vi "Dashboard Main.vi"() -> ()   [LabVIEW 2016]
uses:
  <vilib>/Utility/miscctls.llb/LVRowAndColumnTypeDef.ctl
  <vilib>/event_ctls.llb/eventvkey.ctl
  <vilib>/Rock Robotics/Network Tables/NT Read Boolean.vi
  <vilib>/Rock Robotics/Network Tables/NT Read Numeric Array.vi
  <vilib>/Rock Robotics/WPI/Dashboard/WPI_DashboardLogging Global.vi
panel:
  in  "Camera Settings Right":T1={"Frame Rate"=30, "Compression"=30, "Size"=1, "DB Camera Config"=FALSE} {"Frame Rate" scale=1.0..30.0; "Compression" scale=100.0..-1.0; "Size" items=["640x480", "320x240", "160x120"]}
  in  "Camera Name Right":string(combo)="No Camera Selection"
  out "Camera Info":cluster{"Mbps LED":bool, "Mbps":dbl, "fps":dbl} {"fps" format="%#.1g"; "Mbps" format="%#.1g"}
  in  "Camera Settings":T1={"Frame Rate"=30, "Compression"=30, "Size"=1, "DB Camera Config"=FALSE} {"Frame Rate" scale=1.0..30.0; "Compression" scale=100.0..-1.0; "Size" items=["640x480", "320x240", "160x120"]}
  in  "TCP":refnum<k5>
  in  "Rec Mode":enum32{"Stop", "Record", "Playback"}(radio)
  out "Robot IP":string
  out "Image Message":string="Timeout in Camera Communications"
  in  "Dashboard Tab":T2(tab)
  out "Accelerometer Z Axis":dbl
  out "Accelerometer Y Axis":dbl
  out "Accelerometer X Axis":dbl
  out "Vision Align":bool
  out "LEFT SPEED VARIABLE FEEDBACK":dbl
  in  "LEFT SPEED VARIABLE":dbl
  out "RIGHT SPEED VARIABLE FEEDBACK":dbl
  in  "RIGHT SPEED VARIABLE":dbl
  in  "Select Auto":string(combo)="Select Autonomous ..."
  out "NT Connection":bool
  out "MotorChart R":cluster{"Numeric":dbl, "Numeric":dbl}(graph)
  out "MotorChart L":cluster{"Numeric":dbl, "Numeric":dbl}(graph)
  out "MotorSliders R":cluster{"MotorSlide1":dbl, "MotorSlide2":dbl} {"MotorSlide2" scale=-1.0..1.0 scale format="%#_2e"; "MotorSlide1" scale=-1.0..1.0 scale format="%#_2e"}
  out "MotorSliders L":cluster{"MotorSlide1":dbl, "MotorSlide2":dbl} {"MotorSlide2" scale=-1.0..1.0 scale format="%#_2e"; "MotorSlide1" scale=-1.0..1.0 scale format="%#_2e"}
  out "Gyro":dbl(knob) scale=0.0..360.0
  out "JS1 Z":dbl(slide) scale=-1.0..1.0 scale format="%#_2e"
  out "JS1 Graph":cluster{"X":dbl, "Y":dbl}[](graph)
  out "JS1 Buttons":T3
  out "JS2 Z":dbl(slide) scale=-1.0..1.0 scale format="%#_2e"
  out "JS2 Graph":cluster{"X":dbl, "Y":dbl}[](graph)
  out "JS2 Buttons":T3
  out "Mode":T4(ring)=enum."Auto Disabled"
  out "RightMotors":dbl
  out "LeftMotors":dbl
  out "Right Y Axis":dbl
  out "Right X Axis":dbl
  out "Left X Axis":dbl
  out "Left Y Axis":dbl
  out "Vision Nothing In Sight":bool
  out "Camera Image Right":T5(plugin-control)
  out "X Average":dbl
  out "Vision Align 2":bool
  in  "DB/String 9":string
  in  "DB/String 8":string
  in  "DB/String 7":string
  in  "DB/String 6":string
  in  "DB/String 5":string
  in  "DB/String 4":string
  in  "DB/String 3":string
  in  "DB/String 2":string
  in  "DB/String 1":string
  in  "DB/String 0":string
  in  "DB/Slider 0":dbl(slide) scale=0.0..5.0
  in  "DB/Slider 1":dbl(slide) scale=0.0..5.0
  in  "DB/Slider 2":dbl(slide) scale=0.0..5.0
  in  "DB/Slider 3":dbl(slide) scale=0.0..5.0
  out "DB/LED 3":bool
  out "DB/LED 2":bool
  out "DB/LED 1":bool
  out "DB/LED 0":bool
  in  "DB/Button 3":bool
  in  "DB/Button 2":bool
  in  "DB/Button 1":bool
  in  "DB/Button 0":bool caption="New Name"
  out "Autonoums Delay FEEDBACK":dbl
  in  "Autonoums Delay":dbl
  out "Vision align Range correction VARIABLE FEEDBACK":dbl
  in  "Vision align Range correction VARIABLE":dbl
  out "Vision align Oscillation correction VARIABLE FEEDBACK":dbl
  in  "Vision align Oscillation correction VARIABLE":dbl
  out "Periodic Gyro forward SPEED VARIABLE FEEDBACK":dbl
  in  "Periodic Gyro forward SPEED VARIABLE":dbl
  out "Autonomos Gyro forward SPEED VARIABLE FEEDBACK":dbl
  in  "Autonomos Gyro forward SPEED VARIABLE":dbl
  in  "Test Slider":dbl(slide) scale=0.0..100.0 scale format="%#_3g"
  in  "On/Off":bool caption="Solenoid"
  in  "Test Name":u16(ring) items=["Select the test to run..."]
  in  "Test Tree":string(tree)
  in  "Motor":cluster{"Value":dbl, "Enable":bool} {"Value" scale=-1.0..1.0 scale format="%#_3g"}
  out "Progress":T6 {"Test Progress" scale=0.0..100.0}
  in  "Rev/Fwd":cluster{"Forward":bool, "Reverse":bool}
  in  "Test Ring":u16(ring) items=["Monochrome", "Color"]
  out "Cmd Status":string
  in  "Execute Command":bool
  in  "Command Params":string[][](table)
  in  "Command Selection":i32(listbox)
  in  "CheckList":i32(listbox)
  out "Tree":string(tree)
  out "Camera Image":T5(plugin-control)
  out "Background":bool
  in  "Camera Name":string(combo)="No Camera Selection"
  # "HW"
  # "HW"
  # "Joysticks"
  # "Drive Motors"
  # "Front"
  # "Right"
  # "Left"
  # "Back"
  # "Should be 0.4"
  # "Should be 0.3"
  # "Should be 0.45"
  # "Should be 0.5"
  # "Should be 0.2"
  # "Should be 0.1"
  # "Should be 1500"
  # "This tab is a great place for autonomous settings and robot-specific values.\nPlace controls and indicators inside this tab and match name to\nDashboard Variables on robot. You can also delete this comment."
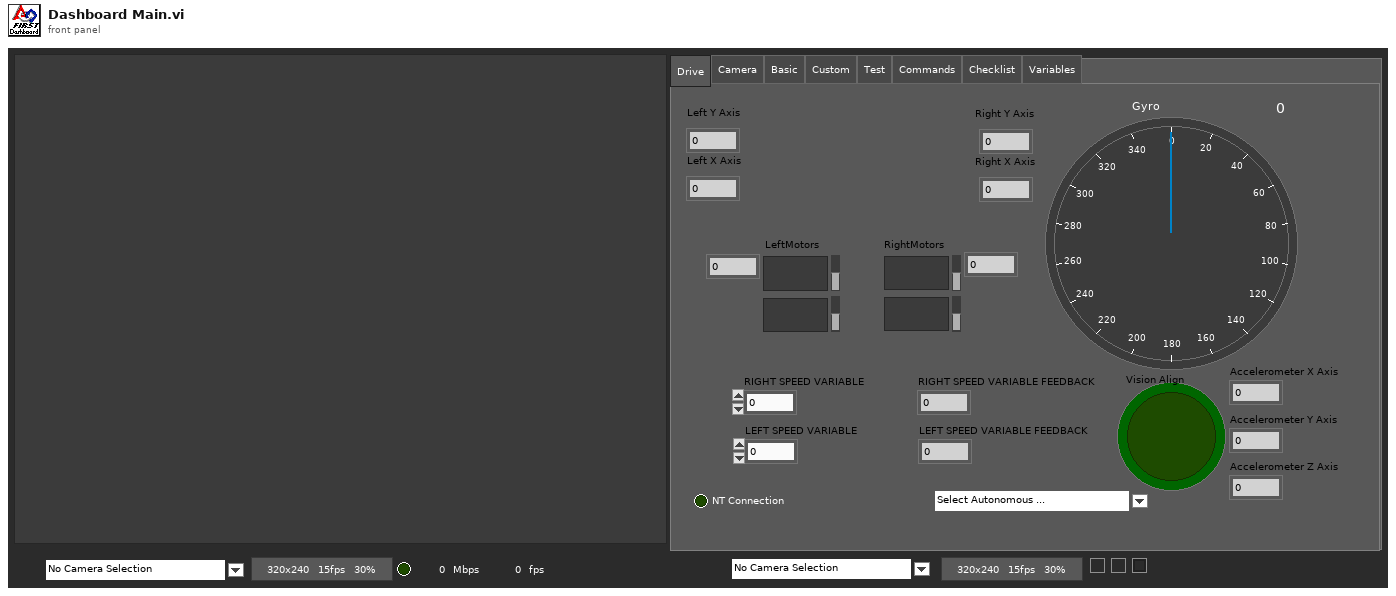
[diagram p1: front panel]
types:
  T1 = cluster{"Frame Rate":i32, "Compression":i32, "Size":u16, "DB Camera Config":bool}
  T2 = enum32{"Drive", "Camera", "Basic", "Custom", "Test", "Commands", "Checklist", "Variables"}
  T3 = cluster{bool, bool, bool, bool, bool, bool, bool, bool, bool, bool, bool, bool}
  T4 = enum8{"Tele-Op Disabled", "Tele-Op Enabled", "Auto Disabled", "Auto Enabled", "Test Disabled", "Test Enabled", "Disconnected", "No Code", "E-Stop"}
  T5 = typedef "IMAQ Image.ctl" = refnum<image>
  T6 = cluster{"Test Progress":u8, "Test Progress Text":string}
  T7 = typedef "Image Type" = u32
  T8 = cluster{"IDs":cluster{"RPC field ID":u16, "Unique ID":u16}, "String":string}
  T9 = enum32{"Drive", "Basic", "Custom", "Test", "Checklist", "Variables"}
  T10 = cluster{"Error Strings":string, "Disable Counts":cluster{u16, u16}, "Rail Faults":cluster{u16, u16, u16}, "Robot IP":string, "DB Mode":u8, "Event Info":cluster{"Name":string, "Type":u8, "Number":u16, "Replay":u8}}
  T11 = cluster{"Storage":cluster{"Disk Free":u64, "RAM Block":u32, "RAM free":u32}, "CPU Utilization":cluster{"CPU % ISR":sgl, "CPU % Time Crit":sgl, "CPU % Timed Str":sgl, "CPU % High":sgl, "CPU % Above":sgl, "CPU % Normal":sgl, "CPU % Low":sgl}, "CAN":cluster{"% Bus Utilization":sgl, "Bus Off Cnt":u32, "TX_FIFO Full Cnt":u32, "Receive Error Cnt":u8, "Transmit Error Cnt":u8}, "HID":cluster{"HID Outputs":u32, "Rumble Low":u16, "Rumble High":u16}[]}
  T12 = cluster{"Status bits":cluster{"Test Mode":bool, "Autonomous":bool, "Enabled":bool, "Code Start":bool, "Brownout":bool, "Reserved 2":bool, "Reserved 3":bool, "E-Stop":bool}, "Code Trace":cluster{"Disabled":bool, "TeleOp":bool, "Auto":bool, "Test":bool}, "Controller Type":enum16{"unknown", "cRIO", "roboRio"}, "Code?":enum16{"unknown", "noCode", "code"}, "Battery V":dbl}
  T13 = cluster{"Control Bits":cluster{"TestMode":bool, "Autonomous":bool, "Enabled":bool, "FMS Present":bool, bool, bool, bool, "E-Stop":bool}, "Team Station ":u8, "Countdown":sgl, "Joystick Values":cluster{"Axes":dbl[], "Buttons":bool[], "POVs":i16[]}[]}
  T14 = cluster{"Axes":dbl[], "Buttons":bool[], "POVs":i16[]}[]
  T15 = cluster{"Axes":dbl[], "Buttons":bool[], "POVs":i16[]}
  T16 = cluster{"Buttons[0]":bool, "Buttons[1]":bool, "Buttons[2]":bool, "Buttons[3]":bool, "Buttons[4]":bool, "Buttons[5]":bool, "Buttons[6]":bool, "Buttons[7]":bool, "Buttons[8]":bool, "Buttons[9]":bool, "Buttons[10]":bool, "Buttons[11]":bool}
  T17 = cluster{"Camera Image":refnum<vi>, "Dashboard Tab":refnum<vi>, "Background":refnum<vi>, "Rec Mode":refnum<vi>, "Test Slider":refnum<vi>, "On/Off ":refnum<vi>, "Test Ring":refnum<vi>, "Rev/Fwd":refnum<vi>, "Test Name":refnum<vi>, "Motor":refnum<vi>, "Progress":refnum<vi>, "CheckList":refnum<vi>, "Tree":refnum<vi>, "Test Tree":refnum<vi>, "Command Params":refnum<vi>, "Command Selection":refnum<vi>, "Execute Command":refnum<vi>, "Cmd Status":refnum<vi>, "Camera Settings":refnum<vi>, "Camera Name":refnum<vi>, "Camera Info":refnum<vi>, "Camera Settings Right":refnum<vi>, "Camera Name Right":refnum<vi>, "Camera Image Right":refnum<vi>}
  T18 = cluster{"Pixels ":cluster{"Start":cluster{"X":dbl, "Y":dbl}, "End":cluster{"X":dbl, "Y":dbl}}, "Real World":cluster{"Start":cluster{"X":dbl, "Y":dbl}, "End":cluster{"X":dbl, "Y":dbl}}}
  T19 = cluster{"Operation":enum16{"Update", "Clear"}, "Color Box":u32}[]
  T20 = typedef "eventvkey.ctl" = enum16{"ASCII", "Enter", "Return", "Shift", "Ctrl", "Alt", "Cmd", "Opt", "Caps", "NumLock", "Clear", "Break", "Up", "Down", "Left", "Right", "Insert", "Delete", "Home", "End", "PageUp", "PageDown", "Escape", "Help", "Pause", "ScrollLock", "F1", "F2", "F3", "F4", "F5", "F6", "F7", "F8", "F9", "F10", "F11", "F12", "F13", "F14", "F15", "F16", "F17", "F18", "F19", "F20", "F21", "F22", "F23", "F24", "Play", "VolumeUp", "VolumeDown", "Mute", "Two Byte Char"}
  T21 = cluster{"Image Size":bool, "Image Type":bool, "Pixel Value":bool, "ROI Information":bool, "Zoom Factor":bool}
  T22 = cluster{"Operation":enum16{"Update", "Clear"}, "Color Box":u32}
  T23 = typedef "LVRowAndColumnTypeDef.ctl" = cluster{"Row":i32, "Column":i32}
  T24 = cluster{"Shift":bool, "Ctrl":bool, "Alt":bool, "Cmd":bool, "Opt":bool}
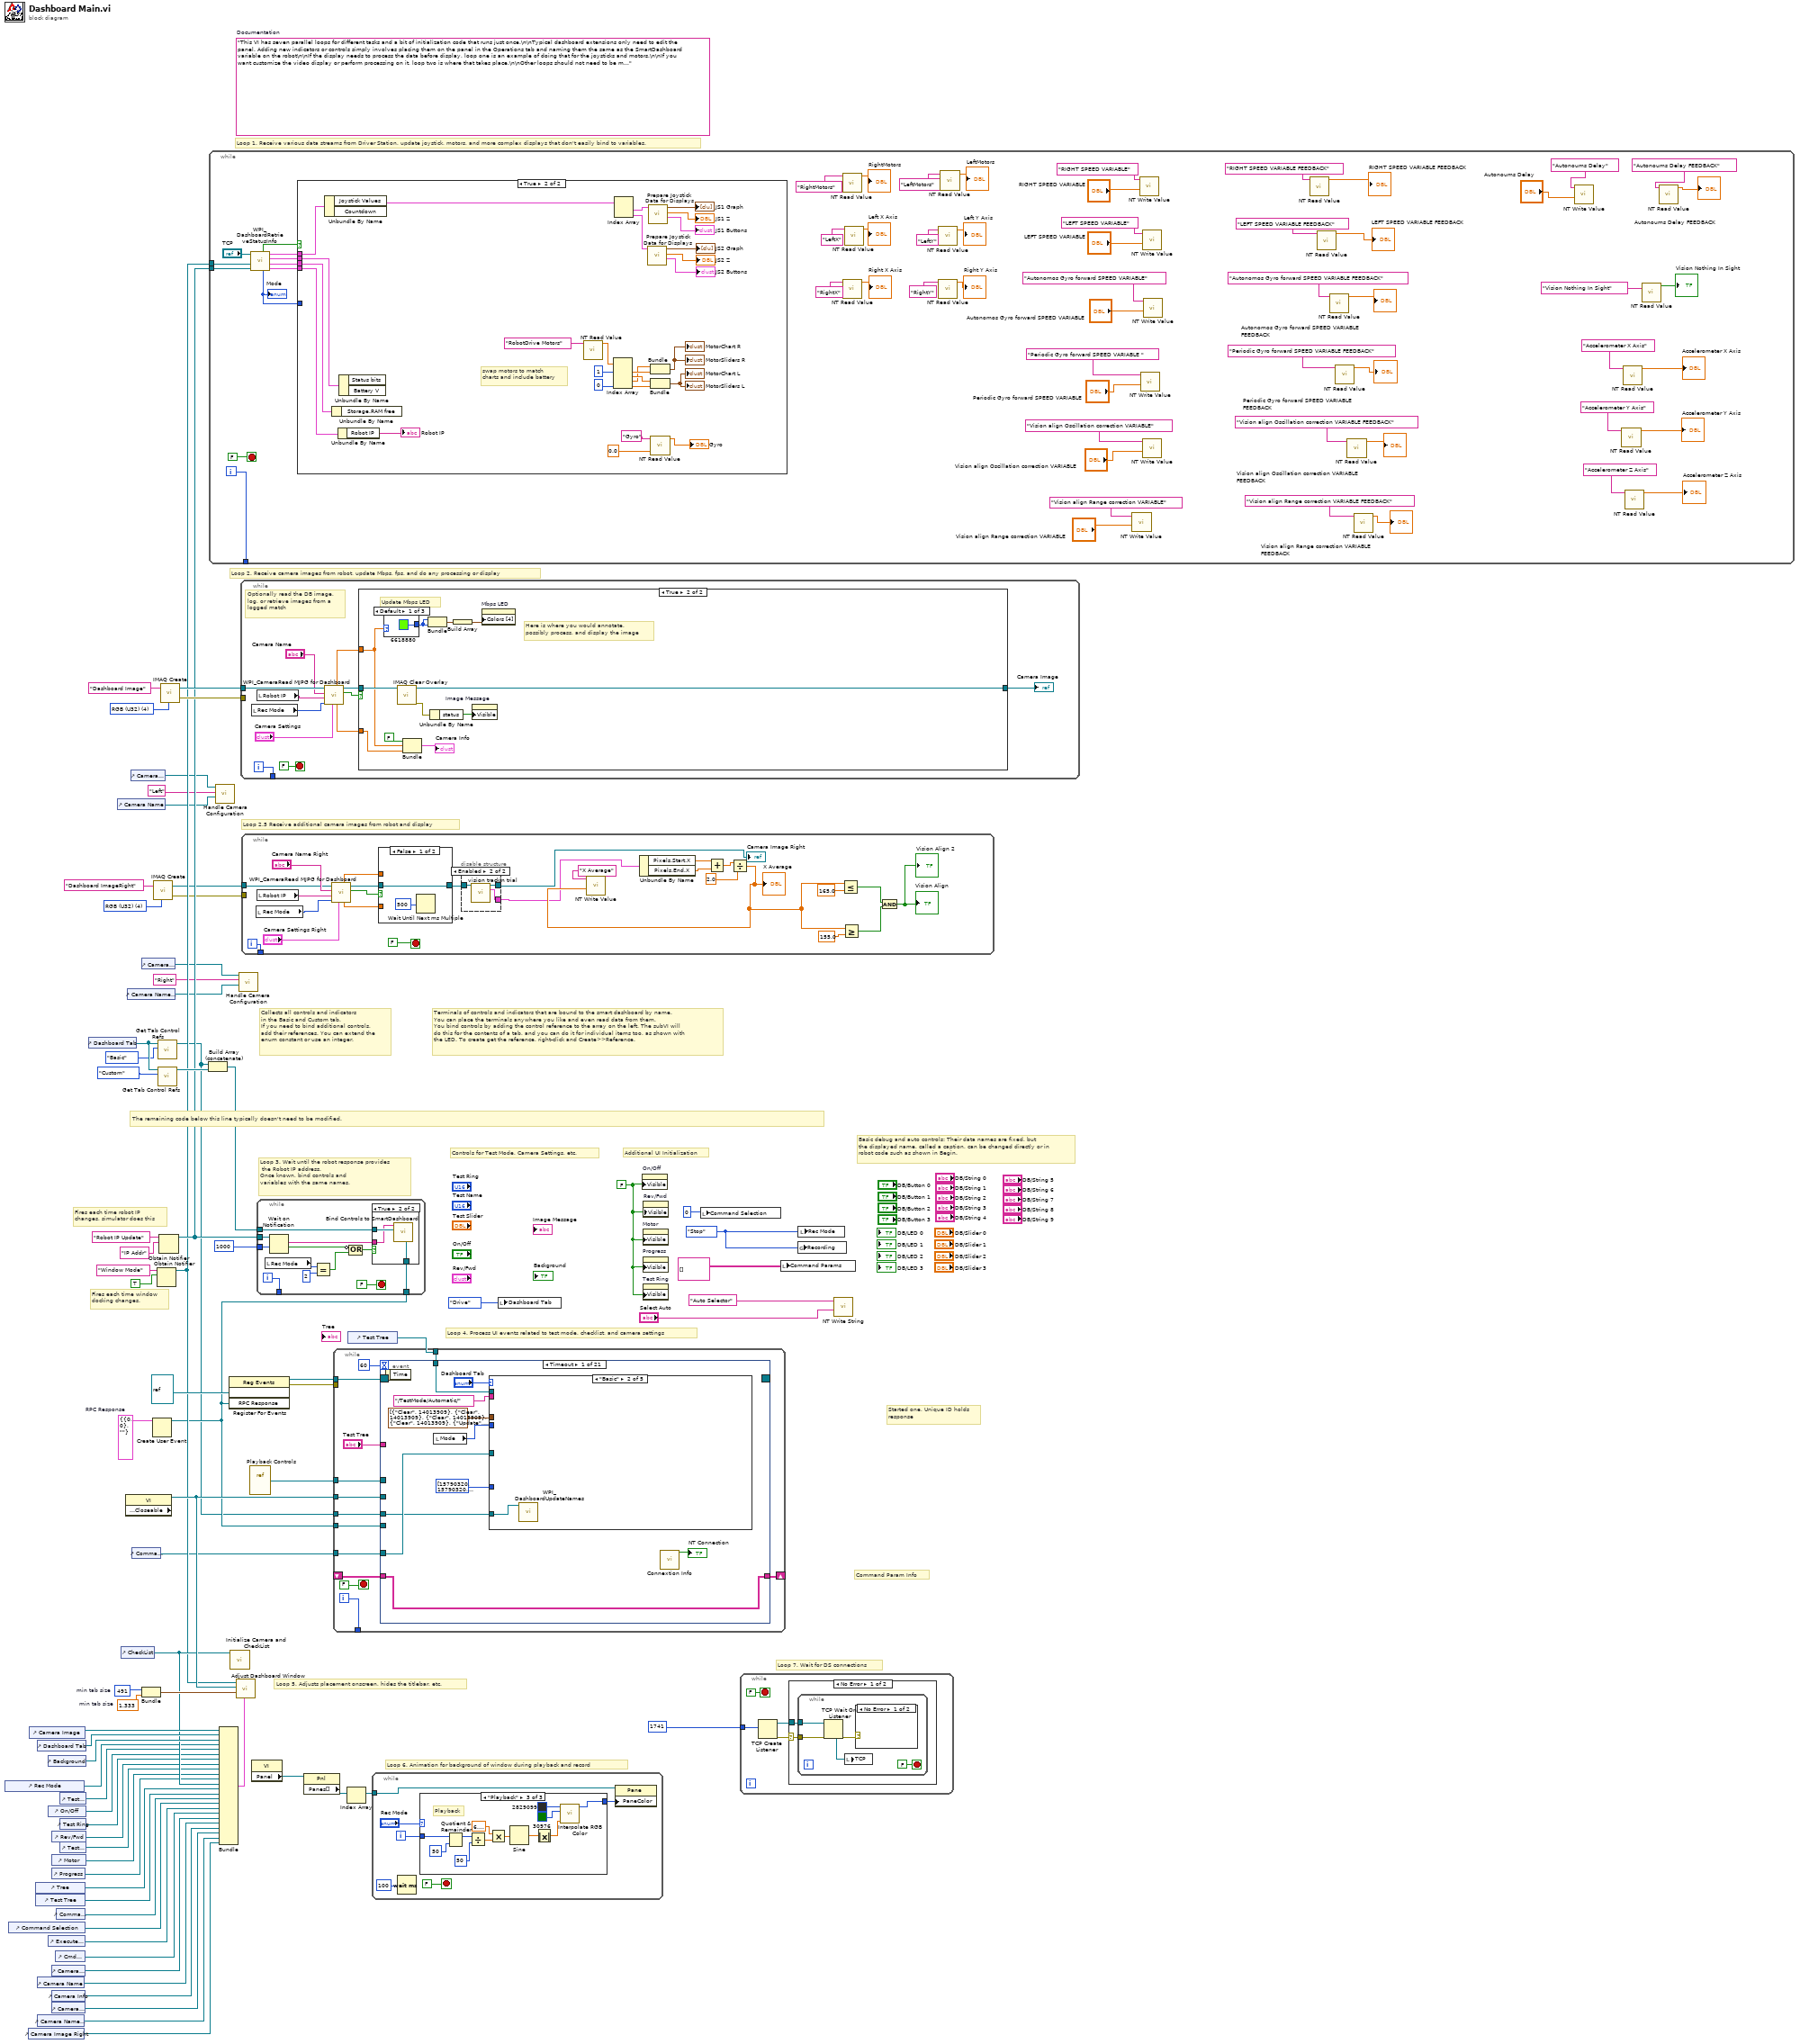
[diagram p0: block diagram]
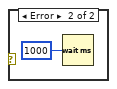
[diagram p4: hidden frame]
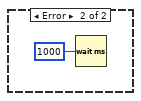
[diagram p5: hidden frame]
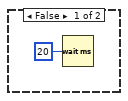
[diagram p6: hidden frame]
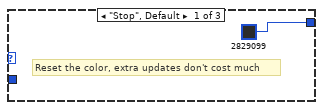
[diagram p7: hidden frame]
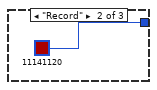
[diagram p8: hidden frame]
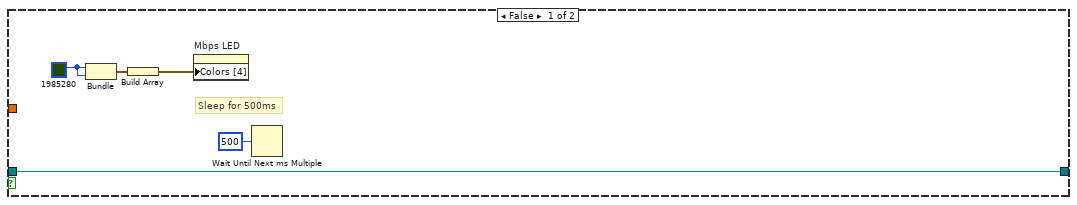
[diagram p10: hidden frame]
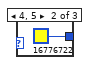
[diagram p11: hidden frame]
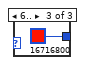
[diagram p12: hidden frame]
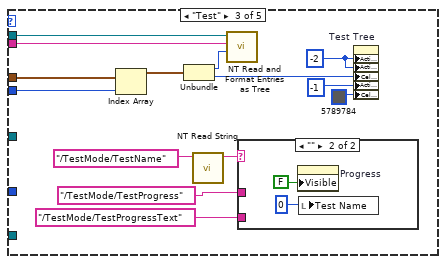
[diagram p14: hidden frame]
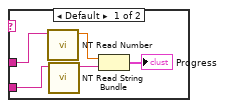
[diagram p15: hidden frame]
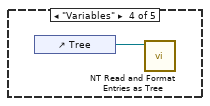
[diagram p16: hidden frame]
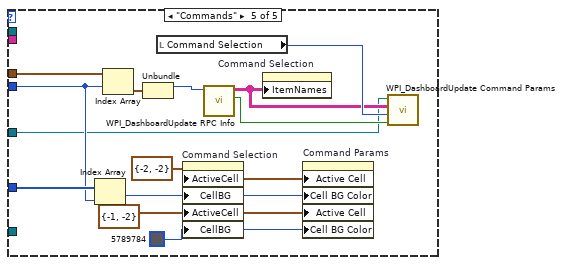
[diagram p17: hidden frame]
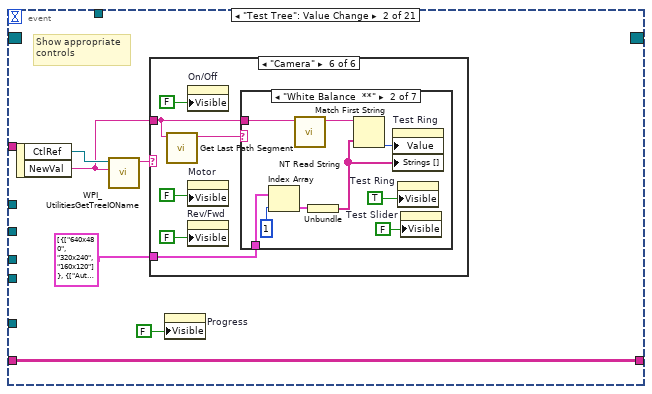
[diagram p18: hidden frame]
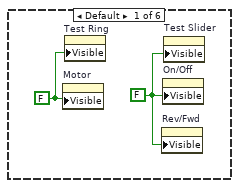
[diagram p19: hidden frame]
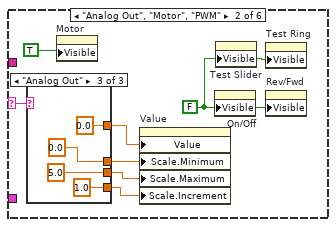
[diagram p20: hidden frame]
diagram:
  w10 = T7 4 items=["Grayscale (U8)", "Grayscale (I16)", "Grayscale (SGL)", "Complex (CSG)", "RGB (U32)", "HSL (U32)", "RGB (U64)"] ("Image Type")
  w26 = T8 {"IDs"={"RPC field ID"=0, "Unique ID"=0}, "String"=""}  # RPC Response
  w51 = 491  # min tab size
  w50 = 1.333  # min tab size
  w58 = enum32{"Stop", "Record", "Playback"}."Stop" ("Rec Mode")
  w33 = FALSE ("Visible")
  (unwired) "This VI has seven parallel loops for different tasks and a bit of initialization code that runs just once.\n\nTypical dashboard extensions only need to edit the panel. Adding new indicators or controls simply involves placing them on the panel in the Operations tab and naming them the same as the SmartDashboard variable on the robot\n\nIf the display needs to process the data before display, loop one is an example of doing that for the joysticks and motors.\n\nIf you want customize the video display or perform processing on it, loop two is where that takes place.\n\nOther loops should not need to be modified. They are pretty standard, and document the task they perform."  # Documentation
  w75 = T7 4 items=["Grayscale (U8)", "Grayscale (I16)", "Grayscale (SGL)", "Complex (CSG)", "RGB (U32)", "HSL (U32)", "RGB (U64)"] ("Image Type")
  # "Loop 2.5 Receive additional camera images from robot and display"
  # "Command Param Info"
  # "Started one, Unique ID holds\nresponse"
  # "Loop 7. Wait for DS connections"
  # "Basic debug and auto controls: Their data names are fixed, but\nthe displayed name, called a caption, can be changed directly or in\nrobot code such as shown in Begin."
  # "Controls for Test Mode, Camera Settings, etc."
  # "Additional UI Initialization"
  # "Loop 6. Animation for background of window during playback and record"
  # "Fires each time robot IP\nchanges, simulator does this"
  # "Fires each time window\ndocking changes."
  # "Collects all controls and indicators\nin the Basic and Custom tab.\nIf you need to bind additional controls,\nadd their references. You can extend the\nenum constant or use an integer."
  # "The remaining code below this line typically doesn't need to be modified."
  # "Loop 4. Process UI events related to test mode, checklist, and camera settings"
  # "Terminals of controls and indicators that are bound to the smart dashboard by name.\nYou can place the terminals anywhere you like and even read data from them.\nYou bind controls by adding the control reference to the array on the left. The subVI will\ndo this for the contents of a tab, and you can do it for individual items too, as shown with\nthe LED. To create get the reference, right-click and Create>>Reference."
  # "Loop 3. Wait until the robot response provides\n the Robot IP address.\nOnce known, bind controls and\nvariables with the same names."
  # "Loop 5. Adjusts placement onscreen, hides the titlebar, etc."
  # "Loop 1. Receive various data streams from Driver Station, update joystick, motors, and more complex displays that don't easily bind to variables."
  # "Loop 2. Receive camera images from robot, update Mbps, fps, and do any processing or display"
  n1 = control-ref of="Rec Mode"() -> (w39:refnum<vi>)
  n2 = control-ref of="Command Selection"() -> (w25:refnum<vi>)
  n3 = control-ref of="Camera Image Right"() -> (w1:refnum<vi>)
  n4 = control-ref of="Camera Image"() -> (w53:refnum<vi>)
  n5 = control-ref of="Tree"() -> (w43:refnum<vi>)
  n6 = control-ref of="Test Tree"() -> (w42:refnum<vi>)
  n7 = control-ref of="Dashboard Tab"() -> (w52:refnum<vi>)
  n8 = control-ref of="Camera Name"() -> (w16:refnum<vi>)
  n9 = control-ref of="Camera Name Right"() -> (w2:refnum<vi>)
  n10 = control-ref of="Execute Command"() -> (w27:refnum<vi>)
  n11 = control-ref of="Background"() -> (w48:refnum<vi>)
  n12 = control-ref of="On/Off"() -> (w37:refnum<vi>)
  n13 = control-ref of="Progress"() -> (w34:refnum<vi>)
  n14 = control-ref of="Camera Settings"() -> (w17:refnum<vi>)
  n15 = control-ref of="Camera Info"() -> (w15:refnum<vi>)
  n16 = control-ref of="Camera Settings Right"() -> (w3:refnum<vi>)
  n17 = control-ref of="Rev/Fwd"() -> (w35:refnum<vi>)
  n18 = control-ref of="Motor"() -> (w40:refnum<vi>)
  n19 = control-ref of="Cmd Status"() -> (w21:refnum<vi>)
  n20 = control-ref of="Command Params"() -> (w28:refnum<vi>)
  n21 = control-ref of="Test Slider"() -> (w38:refnum<vi>)
  n22 = control-ref of="Test Ring"() -> (w36:refnum<vi>)
  n23 = control-ref of="Test Name"() -> (w41:refnum<vi>)
  n24 = control-ref of="Dashboard Tab"() -> (w56:refnum<vi>)
  n25 = control-ref of="Camera Name"() -> (w18:refnum<vi>)
  n26 = control-ref of="CheckList"() -> (w44:refnum<vi>)
  n27 = property class="VI" props=["Front Panel.Closeable"]() -> (reference out=w57:refnum<vi>)  [unwired: 2 in, 2 out]
  n28 = control-ref of="Camera Name Right"() -> (w6:refnum<vi>)
  n29 = control-ref of="Camera Settings"() -> (w19:refnum<vi>)
  n30 = control-ref of="Command Params"() -> (w20:refnum<vi>)
  n31 = control-ref of="Camera Settings Right"() -> (w7:refnum<vi>)
  n32 = Bundle("min tab size"=w51, "min tab size"=w50) -> (w49:cluster{"min tab size":i32, "min tab size":dbl})  [unwired: 1 in]
  n33 = Create User Event(user event datatype=w26) -> (user event=w22:refnum<user-event>)  [unwired: 1 in, 1 out]
  n34 = call "IMAQ Create"("Image Name"="Dashboard ImageRight", "Image Type"=w10) -> ("New Image"=w9:T5, "error out"=w8:errorcluster)  [unwired: 2 in, 1 out]
  n35 = Obtain Notifier(name (unnamed)="Window Mode", notification data type=TRUE) -> (notifier out=w31:refnum<notifier>)  [unwired: 2 in, 2 out]
  n36 = call <vilib>:"Get Tab Control Refs.vi"("Page Index"=T9."Basic" ("Dashboard Tab"), "TabControl in"=w56) -> ("ControlsOnPage"=w14:refnum<vi>[])  [unwired: 9 in]
  n37 = call <vilib>:"Get Tab Control Refs.vi"("Page Index"=T9."Custom" ("Dashboard Tab"), "TabControl in"=w56) -> ("ControlsOnPage"=w55:refnum<vi>[])  [unwired: 9 in]
  n38 = Obtain Notifier(name (unnamed)="Robot IP Update", notification data type="IP Addr" ("name (unnamed)")) -> (notifier out=w32:refnum<notifier>)  [unwired: 2 in, 2 out]
  n39 = call "IMAQ Create"("Image Name"="Dashboard Image", "Image Type"=w75) -> ("New Image"=w73:T5, "error out"=w72:errorcluster)  [unwired: 2 in, 1 out]
  n40 = Build Array (concatenate)(w14, w55) -> (w54:refnum<vi>[])
  n41 = while {
    tunnel: [w133] -> _
    tunnel: w32 -> [w127]
    tunnel: w31 -> [w124]
    i -> [w133]
    stop <- FALSE stop-if-true
    n42 = call <vilib>:"WPI_DashboardRetrieveStatusInfo.vi"("Binding Refnum"=w127, "Window Mode Notifier"=w124, "TCP Cnx"="TCP") -> ("Power and Errors"=w128:T10, "Robot Metrics"=w131:T11, "Status Info"=w132:T12, "Control Info"=w129:T13, "Robot Mode"=w126:T4, "Process?"=w130:bool)  [unwired: 3 in]
    "Mode" <- w126
    n43 = case shown="True" w130 {
      tunnel: w132 -> [_ w162]
      tunnel: w131 -> [_ w161]
      tunnel: w129 -> [_ w160]
      tunnel: w128 -> [_ w159]
      tunnel: w126 -> [_ _]
      frame False {
        n44 = Wait (ms)(milliseconds to wait=u32 20) -> ()  [unwired: 1 out]
      }
      frame True {
        # "swap motors to match\ncharts and include battery"
        n45 = Unbundle By Name(w160) -> ("Joystick Values"=w150:T14)  [unwired: 1 out]
        n46 = Unbundle By Name(w161) -> ()  [unwired: 1 out]
        n47 = Unbundle By Name(w159) -> ("Robot IP"=→"Robot IP":string)
        n48 = Unbundle By Name(w162) -> ()  [unwired: 2 out]
        n49 = call-poly <vilib>:"NT Read Value.vi"("Name"="RobotDrive Motors") -> ("Numeric Array"=w140:dbl[])  [unwired: 9 in, 1 out]
        n50 = Index Array(array=w140, index #1=1, index #4=0) -> (element #1=w154:dbl, element #2=w155:dbl, element #3=w153:dbl, element #4=w158:dbl)  [unwired: 2 in]
        n51 = Index Array(array=w150) -> (element #1=w149:T15, element #2=w145:T15)  [unwired: 2 in]
        n52 = call "Prepare Joystick Data for Displays.vi"("Joystick Values"=w145) -> ("Buttons"=→"JS2 Buttons":T16, "Z Axis"=→"JS2 Z":dbl, "Cartesian Data"=→"JS2 Graph":cluster{"X axis":dbl, "X axis":dbl}[])  [unwired: 8 in]
        n53 = call "Prepare Joystick Data for Displays.vi"("Joystick Values"=w149) -> ("Buttons"=→"JS1 Buttons":T16, "Z Axis"=→"JS1 Z":dbl, "Cartesian Data"=→"JS1 Graph":cluster{"X axis":dbl, "X axis":dbl}[])  [unwired: 8 in]
        n54 = Bundle("Numeric"=w153, "Numeric"=w154) -> (→"MotorChart R" →"MotorSliders R":cluster{"Numeric":dbl, "Numeric":dbl})  [unwired: 1 in]
        n55 = Bundle("Numeric"=w155, "Numeric"=w158) -> (→"MotorChart L" →"MotorSliders L":cluster{"Numeric":dbl, "Numeric":dbl})  [unwired: 1 in]
        n56 = call-poly <vilib>:"NT Read Value.vi"("Default Value"=0.0, "Name"="Gyro") -> ("Numeric"=→"Gyro":dbl)  [unwired: 8 in, 1 out]
      }
    }
    n57 = call-poly <vilib>:"NT Read Value.vi"("Name"="RightMotors") -> ("Numeric"=→"RightMotors":dbl)  [unwired: 9 in, 1 out]
    n58 = call-poly <vilib>:"NT Read Value.vi"("Name"="RightX") -> ("Numeric"=→"Right X Axis":dbl)  [unwired: 9 in, 1 out]
    n59 = call-poly <vilib>:"NT Read Value.vi"("Name"="LeftX") -> ("Numeric"=→"Left X Axis":dbl)  [unwired: 9 in, 1 out]
    n60 = call-poly <vilib>:"NT Read Value.vi"("Name"="LeftY") -> ("Numeric"=→"Left Y Axis":dbl)  [unwired: 9 in, 1 out]
    n61 = call-poly <vilib>:"NT Read Value.vi"("Name"="RightY") -> ("Numeric"=→"Right Y Axis":dbl)  [unwired: 9 in, 1 out]
    n62 = call-poly <vilib>:"NT Read Value.vi"("Name"="LeftMotors") -> ("Numeric"=→"LeftMotors":dbl)  [unwired: 9 in, 1 out]
    n63 = call-poly <vilib>:"NT Write Value.vi"("Numeric"="Vision align Range correction VARIABLE", "Name"="Vision align Range correction VARIABLE") -> ()  [unwired: 9 in, 1 out]
    n64 = call-poly <vilib>:"NT Write Value.vi"("Numeric"="RIGHT SPEED VARIABLE", "Name"="RIGHT SPEED VARIABLE") -> ()  [unwired: 9 in, 1 out]
    n65 = call-poly <vilib>:"NT Write Value.vi"("Numeric"="Periodic Gyro forward SPEED VARIABLE", "Name"="Periodic Gyro forward SPEED VARIABLE ") -> ()  [unwired: 9 in, 1 out]
    n66 = call-poly <vilib>:"NT Write Value.vi"("Numeric"="LEFT SPEED VARIABLE", "Name"="LEFT SPEED VARIABLE") -> ()  [unwired: 9 in, 1 out]
    n67 = call-poly <vilib>:"NT Write Value.vi"("Numeric"="Vision align Oscillation correction VARIABLE", "Name"="Vision align Oscillation correction VARIABLE") -> ()  [unwired: 9 in, 1 out]
    n68 = call-poly <vilib>:"NT Write Value.vi"("Numeric"="Autonomos Gyro forward SPEED VARIABLE", "Name"="Autonomos Gyro forward SPEED VARIABLE") -> ()  [unwired: 9 in, 1 out]
    n69 = call-poly <vilib>:"NT Read Value.vi"("Name"="RIGHT SPEED VARIABLE FEEDBACK") -> ("Numeric"=→"RIGHT SPEED VARIABLE FEEDBACK":dbl)  [unwired: 9 in, 1 out]
    n70 = call-poly <vilib>:"NT Read Value.vi"("Name"="LEFT SPEED VARIABLE FEEDBACK") -> ("Numeric"=→"LEFT SPEED VARIABLE FEEDBACK":dbl)  [unwired: 9 in, 1 out]
    n71 = call-poly <vilib>:"NT Read Value.vi"("Name"="Autonomos Gyro forward SPEED VARIABLE FEEDBACK") -> ("Numeric"=→"Autonomos Gyro forward SPEED VARIABLE FEEDBACK":dbl)  [unwired: 9 in, 1 out]
    n72 = call-poly <vilib>:"NT Read Value.vi"("Name"="Periodic Gyro forward SPEED VARIABLE FEEDBACK") -> ("Numeric"=→"Periodic Gyro forward SPEED VARIABLE FEEDBACK":dbl)  [unwired: 9 in, 1 out]
    n73 = call-poly <vilib>:"NT Read Value.vi"("Name"="Vision align Oscillation correction VARIABLE FEEDBACK") -> ("Numeric"=→"Vision align Oscillation correction VARIABLE FEEDBACK":dbl)  [unwired: 9 in, 1 out]
    n74 = call-poly <vilib>:"NT Read Value.vi"("Name"="Vision align Range correction VARIABLE FEEDBACK") -> ("Numeric"=→"Vision align Range correction VARIABLE FEEDBACK":dbl)  [unwired: 9 in, 1 out]
    n75 = call-poly <vilib>:"NT Write Value.vi"("Numeric"="Autonoums Delay", "Name"="Autonoums Delay") -> ()  [unwired: 9 in, 1 out]
    n76 = call-poly <vilib>:"NT Read Value.vi"("Name"="Accelerometer Y Axis") -> ("Numeric"=→"Accelerometer Y Axis":dbl)  [unwired: 9 in, 1 out]
    n77 = call-poly <vilib>:"NT Read Value.vi"("Name"="Accelerometer X Axis") -> ("Numeric"=→"Accelerometer X Axis":dbl)  [unwired: 9 in, 1 out]
    n78 = call-poly <vilib>:"NT Read Value.vi"("Name"="Accelerometer Z Axis") -> ("Numeric"=→"Accelerometer Z Axis":dbl)  [unwired: 9 in, 1 out]
    n79 = call-poly <vilib>:"NT Read Value.vi"("Name"="Vision Nothing In Sight") -> ("Boolean"=→"Vision Nothing In Sight":bool)  [unwired: 9 in, 1 out]
    n80 = call-poly <vilib>:"NT Read Value.vi"("Name"="Autonoums Delay FEEDBACK") -> ("Numeric"=→"Autonoums Delay FEEDBACK":dbl)  [unwired: 9 in, 1 out]
  }
  n81 = call "Handle Camera Configuration.vi"("CameraNameRef"=w18, "Camera File Name"="Left", "ClusterRef"=w19) -> ()  [unwired: 9 in]
  n82 = Bundle("Camera Image"=w53, "Dashboard Tab"=w52, "Background"=w48, "Rec Mode"=w39, "Test Slider"=w38, "On/Off"=w37, "Test Ring"=w36, "Rev/Fwd"=w35, "Test Name"=w41, "Motor"=w40, "Progress"=w34, "CheckList"=w44, "Tree"=w43, "Test Tree"=w42, "Command Params"=w28, "Command Selection"=w25, "Execute Command"=w27, "Cmd Status"=w21, "Camera Settings"=w17, "Camera Name"=w16, "Camera Info"=w15, "Camera Settings Right"=w3, "Camera Name Right"=w2, "Camera Image Right"=w1) -> (w45:T17)  [unwired: 1 in]
  n83 = register-events(refnum<vi> refnum, w22) -> (reference out=w62:refnum<event-registration>, error out=w61:errorcluster)  [unwired: 2 in]
  n84 = call "Initialize Camera and CheckList.vi"("ListBox in"=w44) -> ()  [unwired: 11 in]
  n85 = call "Adjust Dashboard Window.vi"("Sizing Refnums"=w45, "Size Constraints"=w49, "VI"=w57, "WIn Mode"=w31) -> ()  [unwired: 8 in]
  n86 = call "Handle Camera Configuration.vi"("CameraNameRef"=w6, "Camera File Name"="Right", "ClusterRef"=w7) -> ()  [unwired: 9 in]
  n87 = while {
    tunnel: w73 -> [w172]
    tunnel: w72 -> [_]
    tunnel: [w173] -> _
    i -> [w173]
    stop <- FALSE stop-if-true
    # "Optionally read the DB image,\nlog, or retrieve images from a\nlogged match"
    n88 = local read "Rec Mode"() -> (w168:enum32{"Stop", "Record", "Playback"})
    n89 = local read "Robot IP"() -> (w167:string)
    n90 = call <vilib>:"WPI_CameraRead MJPG for Dashboard.vi"("Camera Settings"="Camera Settings", "Rec Mode"=w168, "Robot IP"=w167, "Camera Name"="Camera Name", "Refnum in"=w172) -> ("Active"=w170:bool, "Refnum out"=w171:T5, "FPS"=w169:dbl, "Bandwidth (Mbps)"=w166:dbl)  [unwired: 3 in]
    n91 = case shown="True" w170 {
      tunnel: w171 -> [w175 w186]
      tunnel: w166 -> [_ w183]
      tunnel: w169 -> [_ w184]
      tunnel: [w175 w180] -> w163
      frame False {
        w177 = u32 1985280 ("Color Box")
        # "Sleep for 500ms"
        n92 = Bundle("Color Box"=w177, "Color Box"=w177) -> (w178:cluster{"Color Box":u32, "Color Box":u32})  [unwired: 1 out]
        n93 = Build Array(w178) -> (w176:cluster{"Color Box":u32, "Color Box":u32}[])
        n94 = property on="Mbps LED" class="Bool (strict)"("Colors [4]"=w176) -> ()  [unwired: 2 in, 2 out]
        n95 = Wait Until Next ms Multiple(millisecond multiple=u32 500) -> ()  [unwired: 1 out]
      }
      frame True {
        # "Here is where you would annotate,\npossibly process, and display the image"
        # "Update Mbps LED"
        n96 = case shown="Default" w183 {
          tunnel: [u32 6618880 ("Color Box") u32 16776722 ("Color Box") u32 16716800 ("Color Box")] -> w187
          frame Default {
          }
          frame 4, 5 {
          }
          frame 6.. {
          }
        }
        n97 = call "IMAQ Clear Overlay"("Image"=w186) -> ("error out"=w189:errorcluster, "Image Out"=w180:T5)  [unwired: 2 in, 7 out]
        n98 = Bundle(FALSE, "Bandwidth (Mbps)"=w183, "FPS"=w184) -> (→"Camera Info":cluster{bool, "Bandwidth (Mbps)":dbl, "FPS":dbl})  [unwired: 1 in]
        n99 = Bundle("Color Box"=w187, "Color Box"=w187) -> (w188:cluster{"Color Box":u32, "Color Box":u32})  [unwired: 1 out]
        n100 = Unbundle By Name(w189) -> ("status"=w190:bool)
        n101 = Build Array(w188) -> (w185:cluster{"Color Box":u32, "Color Box":u32}[])
        n102 = property on="Image Message" class="Str"("Visible"=w190) -> ()  [unwired: 2 in, 2 out]
        n103 = property on="Mbps LED" class="Bool (strict)"("Colors [4]"=w185) -> ()  [unwired: 2 in, 2 out]
      }
    }
    "Camera Image" <- w163
  }
  n104 = while {
    tunnel: w9 -> [w217]
    tunnel: w8 -> [_]
    tunnel: [w211] -> _
    i -> [w211]
    stop <- FALSE stop-if-true
    n105 = local read "Rec Mode"() -> (w215:enum32{"Stop", "Record", "Playback"})
    n106 = local read "Robot IP"() -> (w216:string)
    n107 = call <vilib>:"WPI_CameraRead MJPG for Dashboard.vi"("Camera Settings"="Camera Settings Right", "Rec Mode"=w215, "Robot IP"=w216, "Camera Name"="Camera Name Right", "Refnum in"=w217) -> ("Active"=w210:bool, "Refnum out"=w213:T5, "FPS"=w208:dbl, "Bandwidth (Mbps)"=w209:dbl)  [unwired: 3 in]
    n108 = case shown="False" w210 {
      tunnel: w213 -> [w222 w224]
      tunnel: w209 -> [_ _]
      tunnel: w208 -> [_ _]
      tunnel: [w222 w224] -> w197
      frame False {
        n109 = Wait Until Next ms Multiple(millisecond multiple=u32 500) -> ()  [unwired: 1 out]
      }
      frame True {
      }
    }
    n110 = disable-structure shown="Enabled" {
      disable-tunnel: w197 -> [_ w219]
      disable-tunnel: [_ w221] -> w196
      disable-tunnel: [_ w220] -> w195
      frame Disabled {
      }
      frame Enabled {
        n111 = call "vision trackin trial.vi"("Image In"=w219) -> ("Image Out"=w221:T5, "Clamp Points (Max Clamp 1)"=w220:T18)  [unwired: 23 in, 2 out]
      }
    }
    "Camera Image Right" <- w196
    n112 = Unbundle By Name(w195) -> ("Pixels.Start.X"=w204:dbl, "Pixels.End.X"=w205:dbl)
    n113 = Add(x=w204, y=w205) -> (x+y=w206:dbl)
    n114 = Divide(x=w206, y=2.0) -> (x/y=w202:dbl)
    "X Average" <- w202
    n115 = call-poly <vilib>:"NT Write Value.vi"("Numeric"=w202, "Name"="X Average") -> ()  [unwired: 9 in, 1 out]
    n116 = Less Or Equal?(x=w202, y=165.0) -> (x <= y?=w201:bool)
    n117 = Greater Or Equal?(x=w202, y=155.0) -> (x >= y?=w200:bool)
    n118 = And(x=w201, y=w200) -> (x .and. y?=→"Vision Align" →"Vision Align 2":bool)
  }
  n119 = vi-ref "Playback Controls.vi"() -> (w63:refnum<vi>)
  n120 = property class="VI"() -> ("Panel"=w65:refnum<vi>)  [unwired: 2 in, 2 out]
  n121 = while {
    tunnel: w54 -> [w236]
    tunnel: w32 -> [w234]
    tunnel: [w232] -> _
    tunnel: u32 1000 ("milliseconds to wait") -> [w231]
    tunnel: w22 -> [w225]
    i -> [w232]
    stop <- FALSE stop-if-true
    n122 = local read "Rec Mode"() -> (w227:enum32{"Stop", "Record", "Playback"})
    n123 = Wait on Notification(notifier=w234, timeout in ms (-1)=w231) -> (notification=w233:string, timed out?=w229:bool)  [unwired: 2 in, 2 out]
    n124 = Equal?(x=w227, y=u16 2 ("Rec Mode")) -> (x = y?=w228:bool)
    n125 = Compound Arithmetic op=OR(invert w229, w228) -> (w230:bool)
    n126 = case shown="True" w230 {
      tunnel: w236 -> [_ w239]
      tunnel: w233 -> [_ w238]
      tunnel: w225 -> [_ w237]
      frame False {
      }
      frame True {
        n127 = call <vilib>:"Bind Controls to SmartDashboard.vi"("RPC ref"=w237, "Bound Control Refs"=w239, "Server IP Address"=w238) -> ()  [unwired: 9 in]
      }
    }
  }
  n128 = property class="Pnl"(reference=w65) -> ("Panes[]"=w66:refnum<vi>[])  [unwired: 1 in, 2 out]
  n129 = Index Array(array=w66) -> (element=w64:refnum<vi>)  [unwired: 1 in]
  n130 = control-ref of="Test Tree"() -> (w67:refnum<vi>)
  n131 = while {
    tunnel: [w249] -> _
    tunnel: w67 -> [w248]
    tunnel: w63 -> [w247]
    tunnel: w62 -> [w246]
    tunnel: w61 -> [_]
    tunnel: w57 -> [w245]
    tunnel: w22 -> [w244]
    tunnel: w20 -> [w243]
    shift-right: [w242] -> _
    shift-left: _ -> [w241]
    tunnel: w14 -> [w240]
    i -> [w249]
    stop <- FALSE stop-if-true
    n132 = event shown="[0] Timeout" {
      selector: w246 -> [_ _ _ _ _ _ _ _ _ _ _ _ _ _ _ _ _ _ _ _ _]
      dyn-events: [_ _ _ _ _ _ _ _ _ _ _ _ _ _ _ _ w505 _ _ _ _] -> _
      timeout: u32 60 ("milliseconds to wait") -> [_ _ _ _ _ _ _ _ _ _ _ _ _ _ _ _ _ _ _ _ _]
      tunnel: w248 -> [w261 _ _ _ _ _ _ _ _ _ _ _ _ _ _ _ _ _ _ _ _]
      tunnel: "Test Tree" -> [_ _ _ _ _ _ _ _ _ _ _ w472 w480 w482 w486 w494 _ _ _ _ _]
      tunnel: w247 -> [_ _ _ _ _ _ _ _ _ _ _ _ _ _ _ _ w507 _ w525 _ _]
      tunnel: w245 -> [_ _ _ _ _ _ _ _ _ _ _ _ _ _ _ _ w503 _ _ _ _]
      tunnel: w244 -> [_ _ _ _ _ _ _ _ _ _ _ _ _ _ _ _ w499 _ _ _ _]
      tunnel: w243 -> [w256 _ _ _ _ _ w423 _ _ _ _ _ _ _ _ _ _ _ _ _ _]
      tunnel: [w255 w300 w402 w407 w416 w420 w421 w430 w440 w447 w459 w471 w478 w481 w485 w493 w498 w520 w522 w526 w537] -> w242
      tunnel: w241 -> [w255 w300 w402 w407 w416 w420 w421 _ _ w447 w459 w471 w478 w481 w485 w493 w498 w520 w522 w526 w537]
      tunnel: w240 -> [w253 _ _ _ _ _ _ _ _ _ _ _ _ _ _ _ _ _ _ _ _]
      event Timeout {
        n133 = event-data() -> ()  [unwired: 1 in, 1 out]
        n134 = local read "Mode"() -> (w258:T4)
        n135 = case shown="\"Basic\"" "Dashboard Tab" {
          tunnel: w261 -> [_ _ w277 _ _]
          tunnel: "/TestMode/Automatic/" ("Name Pattern") -> [_ _ w276 _ _]
          tunnel: T19 [{"Operation"=enum."Clear", "Color Box"=14013909}, {"Operation"=enum."Clear", "Color Box"=14013909}, {"Operation"=enum."Clear", "Color Box"=14013909}, {"Operation"=enum."Clear", "Color Box"=14013909}, {"Operation"=enum."Update", "Color Box"=14013909}, {"Operation"=enum."Update", "Color Box"=16777215}, {"Operation"=enum."Clear", "Color Box"=14013909}, {"Operation"=enum."Clear", "Color Box"=14013909}, {"Operation"=enum."Clear", "Color Box"=14013909}] -> [_ _ w269 _ w293]
          tunnel: w258 -> [_ _ w268 _ w292]
          tunnel: u32[] [15790320, 15790320, 15790320, 15790320, 16777215, 16777215, 15790320, 15790320, 15790320] -> [_ _ _ _ w298]
          tunnel: w256 -> [_ _ _ _ w286]
          tunnel: w253 -> [_ w263 _ _ _]
          frame "Custom", Default {
          }
          frame "Basic" {
            n136 = call <vilib>:"WPI_DashboardUpdateNames.vi"("Controls on Tab"=w263) -> ()  [unwired: 11 in]
          }
          frame "Test" {
            w275 = -2 ("Active Item:Row Number")
            n137 = Index Array(array=w269, index=w268) -> (element=w270:T22)
            n138 = Unbundle(w270) -> ("Operation"=w271:enum16{"Update", "Clear"}, "Color Box"=w272:u32)
            n139 = call <vilib>:"NT Read String.vi"("Name"="/TestMode/TestName") -> ("String"=w266:string)  [unwired: 9 in, 1 out]
            n140 = call <vilib>:"NT Read and Format Entries as Tree.vi"("Operation"=w271, "Name Pattern"=w276, "Tree Refnum"=w277) -> ()  [unwired: 7 in, 2 out]
            n141 = case shown="\"\"" w266 {
              tunnel: "/TestMode/TestProgress" ("Name") -> [w279 _]
              tunnel: "/TestMode/TestProgressText" ("Name") -> [w278 _]
              frame Default {
                n142 = call <vilib>:"NT Read Number.vi"("Name"=w279) -> ("Numeric"=w280:dbl)  [unwired: 9 in, 1 out]
                n143 = call <vilib>:"NT Read String.vi"("Name"=w278) -> ("String"=w281:string)  [unwired: 9 in, 1 out]
                n144 = Bundle("Numeric"=w280, "String"=w281) -> (→"Progress":cluster{"Numeric":dbl, "String":string})  [unwired: 1 in]
              }
              frame "" {
                n145 = property on="Progress" class="Clust (strict)"("Visible"=FALSE) -> ()  [unwired: 2 in, 2 out]
                n146 = local write "Test Name"(u16 0) -> ()
              }
            }
            n147 = property on="Test Tree" class="Tree (strict)"("Active Item Row Number"=w275, "ActiveColNum"=w275, "CellBG"=w272, "Active Item Row Number"=-1 ("Active Item:Row Number"), "CellBG"=u32 5789784 ("Color Box")) -> ()  [unwired: 2 in, 2 out]
          }
          frame "Variables" {
            n148 = control-ref of="Tree"() -> (w285:refnum<vi>)
            n149 = call <vilib>:"NT Read and Format Entries as Tree.vi"("Tree Refnum"=w285) -> ()  [unwired: 9 in, 2 out]
          }
          frame "Commands" {
            w294 = u32 5789784 ("Color Box")
            w295 = T23 {"Row"=-1, "Column"=-2} ("Active Cell:Active Cell")
            w297 = T23 {"Row"=-2, "Column"=-2} ("Active Cell:Active Cell")
            n150 = Index Array(array=w298, index=w292) -> (element=w296:u32)
            n151 = Index Array(array=w293, index=w292) -> (element=w291:T22)
            n152 = Unbundle(w291) -> ("Operation"=w290:enum16{"Update", "Clear"})  [unwired: 1 out]
            n153 = local read "Command Selection"() -> (w289:i32)
            n154 = property on="Command Selection" class="MCListbox (strict)"("ActiveCell"=w297, "CellBG"=w296, "ActiveCell"=w295, "CellBG"=w294) -> ()  [unwired: 2 in, 2 out]
            n155 = call <vilib>:"WPI_DashboardUpdate RPC Info.vi"("Operation"=w290) -> ("update"=w288:bool, "commands"=w287:string[][])  [unwired: 9 in]
            n156 = property on="Command Selection" class="MCListbox (strict)"("ItemNames"=w287) -> ()  [unwired: 2 in, 2 out]
            n157 = property on="Command Params" class="Tbl (strict)"("Active Cell"=w297, "Cell BG Color"=w296, "Active Cell"=w295, "Cell BG Color"=w294) -> ()  [unwired: 2 in, 2 out]
            n158 = call <vilib>:"WPI_DashboardUpdate Command Params.vi"("Update"=w288, "NewVal"=w289, "Commands"=w287, "Param Tbl"=w286) -> ()  [unwired: 7 in, 1 out]
          }
        }
        n159 = call <vilib>:"Connextion Info.vi"() -> ("Connected"=→"NT Connection":bool)  [unwired: 10 in, 1 out]
      }
      event "Test Tree": Value Change {
        # "Show appropriate\ncontrols"
        n160 = event-data() -> ("CtlRef"=w303:refnum<vi>, "NewVal"=w301:string)  [unwired: 1 in]
        n161 = call <vilib>:"WPI_UtilitiesGetTreeIOName.vi"("NewVal"=w301, "TreeControl in"=w303) -> ("I/O Name"=w304:string)  [unwired: 9 in]
        n162 = case shown="\"Camera\"" w304 {
          selector: w304 -> [_ w311 _ w333 w342 _]
          tunnel: w301 -> [_ _ w330 w332 _ w349]
          tunnel: cluster{string[]}[] [{["640x480", "320x240", "160x120"]}, {["Auto", "Fixed indoor", "Fixed outdoor 1", "Fixed outdoor 2", "Fixed fluorescent 1", "Fixed fluorescent 2", "Hold current"]}, {["Auto", "Flicker-free 50 Hz", "Flicker-free 60 Hz", "Hold current"]}, {["None", "Prioritize frame rate", "Prioritize image quality"]}, {["Monochrome", "Color"]}] -> [_ _ _ _ _ w348]
          frame Default {
            w306 = FALSE ("Visible")
            w305 = FALSE ("Visible")
            n163 = property on="Motor" class="Clust (strict)"("Visible"=w305) -> ()  [unwired: 2 in, 2 out]
            n164 = property on="Test Ring" class="Ring (strict)"("Visible"=w305) -> ()  [unwired: 2 in, 2 out]
            n165 = property on="Rev/Fwd" class="Clust (strict)"("Visible"=w306) -> ()  [unwired: 2 in, 2 out]
            n166 = property on="On/Off" class="Bool (strict)"("Visible"=w306) -> ()  [unwired: 2 in, 2 out]
            n167 = property on="Test Slider" class="Slide (strict)"("Visible"=w306) -> ()  [unwired: 2 in, 2 out]
          }
          frame "Analog Out", "Motor", "PWM" {
            w312 = FALSE ("Visible")
            n168 = case shown="\"Analog Out\"" w311 {
              tunnel: [1.0 ("Value") -1.0 ("Value") 0.0 ("Value")] -> w310
              tunnel: [255.0 ("Value") 1.0 ("Value") 5.0 ("Value")] -> w309
              tunnel: [128.0 ("Value") 0.0 ("Value") 0.0 ("Value")] -> w308
              tunnel: [64.0 ("Value") 0.5 ("Value") 1.0 ("Value")] -> w307
              frame "PWM" {
              }
              frame "Motor", Default {
              }
              frame "Analog Out" {
              }
            }
            n169 = property on="Motor" class="Clust (strict)"("Visible"=TRUE) -> ()  [unwired: 2 in, 2 out]
            n170 = property on="Value" class="Slide (strict)"("Value"=w308, "Scale.Minimum"=w310, "Scale.Maximum"=w309, "Scale.Increment"=w307) -> ()  [unwired: 2 in, 2 out]
            n171 = property on="On/Off" class="Bool (strict)"("Visible"=w312) -> ()  [unwired: 2 in, 2 out]
            n172 = property on="Test Slider" class="Slide (strict)"("Visible"=w312) -> ()  [unwired: 2 in, 2 out]
            n173 = property on="Test Ring" class="Ring (strict)"("Visible"=w312) -> ()  [unwired: 2 in, 2 out]
            n174 = property on="Rev/Fwd" class="Clust (strict)"("Visible"=w312) -> ()  [unwired: 2 in, 2 out]
          }
          frame "Servo" {
            w328 = FALSE ("Visible")
            n175 = call <vilib>:"NT Read Number.vi"("Name"=w330) -> ("Numeric"=w329:dbl)  [unwired: 9 in, 1 out]
            n176 = property on="Test Slider" class="Slide (strict)"("Visible"=TRUE, "Scale.Maximum"=170.0 ("Scale.Range:Maximum")) -> ()  [unwired: 2 in, 2 out]
            n177 = local write "Test Slider"(w329) -> ()
            n178 = property on="Motor" class="Clust (strict)"("Visible"=w328) -> ()  [unwired: 2 in, 2 out]
            n179 = property on="Rev/Fwd" class="Clust (strict)"("Visible"=w328) -> ()  [unwired: 2 in, 2 out]
            n180 = property on="On/Off" class="Bool (strict)"("Visible"=w328) -> ()  [unwired: 2 in, 2 out]
            n181 = property on="Test Ring" class="Ring (strict)"("Visible"=w328) -> ()  [unwired: 2 in, 2 out]
          }
          frame "Relay", "Solenoid" {
            w331 = FALSE ("Visible")
            n182 = property on="Motor" class="Clust (strict)"("Visible"=w331) -> ()  [unwired: 2 in, 2 out]
            n183 = property on="Test Slider" class="Slide (strict)"("Visible"=w331) -> ()  [unwired: 2 in, 2 out]
            n184 = Search and Replace String(input string=w332, search string="/Value  **", replace string="/Direction") -> (result string=w338:string)  [unwired: 5 in, 3 out]
            n185 = property on="Test Ring" class="Ring (strict)"("Visible"=w331) -> ()  [unwired: 2 in, 2 out]
            n186 = call <vilib>:"NT Read String.vi"("Name"=w338) -> ("String"=w336:string)  [unwired: 9 in, 1 out]
            n187 = Equal?(x="Both directions", y=w336) -> (x = y?=w334:bool)
            n188 = Not(x=w334) -> (.not. x?=w335:bool)
            n189 = property on="Rev/Fwd" class="Clust (strict)"("Visible"=w334) -> ()  [unwired: 2 in, 2 out]
            n190 = property on="On/Off" class="Bool (strict)"("Visible"=w335, "Caption.Text"=w333) -> ()  [unwired: 2 in, 2 out]
          }
          frame "Compressor", "Digital Out" {
            w341 = FALSE ("Visible")
            # "Get direction and finish"
            n191 = property on="Motor" class="Clust (strict)"("Visible"=w341) -> ()  [unwired: 2 in, 2 out]
            n192 = property on="Test Slider" class="Slide (strict)"("Visible"=w341) -> ()  [unwired: 2 in, 2 out]
            n193 = property on="Test Ring" class="Ring (strict)"("Visible"=w341) -> ()  [unwired: 2 in, 2 out]
            n194 = property on="On/Off" class="Bool (strict)"("Visible"=TRUE, "Caption.Text"=w342) -> ()  [unwired: 2 in, 2 out]
            n195 = property on="Rev/Fwd" class="Clust (strict)"("Visible"=FALSE) -> ()  [unwired: 2 in, 2 out]
          }
          frame "Camera" {
            n196 = call <vilib>:"Get Last Path Segment.vi"("String in"=w349) -> ("String out"=w350:string)  [unwired: 10 in]
            n197 = property on="On/Off" class="Bool (strict)"("Visible"=FALSE) -> ()  [unwired: 2 in, 2 out]
            n198 = property on="Motor" class="Clust (strict)"("Visible"=FALSE) -> ()  [unwired: 2 in, 2 out]
            n199 = property on="Rev/Fwd" class="Clust (strict)"("Visible"=FALSE) -> ()  [unwired: 2 in, 2 out]
            n200 = case shown="\"White Balance  **\"" w350 {
              tunnel: w349 -> [w356 w365 w374 w383 w392 _ w398]
              tunnel: w348 -> [w354 w362 w371 w380 w389 _ _]
              frame "Size  **" {
                n201 = Index Array(array=w354) -> (element=w353:cluster{string[]})  [unwired: 1 in]
                n202 = call <vilib>:"NT Read String.vi"("Name"=w356) -> ("String"=w355:string)  [unwired: 9 in, 1 out]
                n203 = Unbundle(w353) -> (w351:string[])
                n204 = Match First String(2:w351, 3:w355) -> (0:w352:i32)  [unwired: 1 out]
                n205 = property on="Test Ring" class="Ring (strict)"("Value"=w352, "Strings []"=w351) -> ()  [unwired: 2 in, 2 out]
                n206 = property on="Test Ring" class="Ring (strict)"("Visible"=TRUE) -> ()  [unwired: 2 in, 2 out]
                n207 = property on="Test Slider" class="Slide (strict)"("Visible"=FALSE) -> ()  [unwired: 2 in, 2 out]
              }
              frame "White Balance  **" {
                n208 = Index Array(array=w362, index=1) -> (element=w363:cluster{string[]})
                n209 = call <vilib>:"NT Read String.vi"("Name"=w365) -> ("String"=w364:string)  [unwired: 9 in, 1 out]
                n210 = Unbundle(w363) -> (w360:string[])
                n211 = Match First String(2:w360, 3:w364) -> (0:w359:i32)  [unwired: 1 out]
                n212 = property on="Test Ring" class="Ring (strict)"("Value"=w359, "Strings []"=w360) -> ()  [unwired: 2 in, 2 out]
                n213 = property on="Test Ring" class="Ring (strict)"("Visible"=TRUE) -> ()  [unwired: 2 in, 2 out]
                n214 = property on="Test Slider" class="Slide (strict)"("Visible"=FALSE) -> ()  [unwired: 2 in, 2 out]
              }
              frame "Exposure  **" {
                n215 = Index Array(array=w371, index=2) -> (element=w372:cluster{string[]})
                n216 = call <vilib>:"NT Read String.vi"("Name"=w374) -> ("String"=w373:string)  [unwired: 9 in, 1 out]
                n217 = Unbundle(w372) -> (w368:string[])
                n218 = Match First String(2:w368, 3:w373) -> (0:w369:i32)  [unwired: 1 out]
                n219 = property on="Test Ring" class="Ring (strict)"("Value"=w369, "Strings []"=w368) -> ()  [unwired: 2 in, 2 out]
                n220 = property on="Test Ring" class="Ring (strict)"("Visible"=TRUE) -> ()  [unwired: 2 in, 2 out]
                n221 = property on="Test Slider" class="Slide (strict)"("Visible"=FALSE) -> ()  [unwired: 2 in, 2 out]
              }
              frame "Exposure Priority  **" {
                n222 = Index Array(array=w380, index=3) -> (element=w381:cluster{string[]})
                n223 = call <vilib>:"NT Read String.vi"("Name"=w383) -> ("String"=w382:string)  [unwired: 9 in, 1 out]
                n224 = Unbundle(w381) -> (w377:string[])
                n225 = Match First String(2:w377, 3:w382) -> (0:w378:i32)  [unwired: 1 out]
                n226 = property on="Test Ring" class="Ring (strict)"("Value"=w378, "Strings []"=w377) -> ()  [unwired: 2 in, 2 out]
                n227 = property on="Test Ring" class="Ring (strict)"("Visible"=TRUE) -> ()  [unwired: 2 in, 2 out]
                n228 = property on="Test Slider" class="Slide (strict)"("Visible"=FALSE) -> ()  [unwired: 2 in, 2 out]
              }
              frame "Color Enable  **" {
                n229 = Index Array(array=w389, index=4) -> (element=w390:cluster{string[]})
                n230 = call <vilib>:"NT Read String.vi"("Name"=w392) -> ("String"=w391:string)  [unwired: 9 in, 1 out]
                n231 = Unbundle(w390) -> (w386:string[])
                n232 = Match First String(2:w386, 3:w391) -> (0:w387:i32)  [unwired: 1 out]
                n233 = property on="Test Ring" class="Ring (strict)"("Value"=w387, "Strings []"=w386) -> ()  [unwired: 2 in, 2 out]
                n234 = property on="Test Ring" class="Ring (strict)"("Visible"=TRUE) -> ()  [unwired: 2 in, 2 out]
                n235 = property on="Test Slider" class="Slide (strict)"("Visible"=FALSE) -> ()  [unwired: 2 in, 2 out]
              }
              frame Default {
                n236 = property on="Test Ring" class="Ring (strict)"("Visible"=FALSE) -> ()  [unwired: 2 in, 2 out]
                n237 = property on="Test Slider" class="Slide (strict)"("Visible"=FALSE) -> ()  [unwired: 2 in, 2 out]
              }
              frame "Brightness  **", "Color Level  **", "Compression  **", "FPS  **", "Sharpness  **" {
                n238 = call <vilib>:"NT Read Number.vi"("Name"=w398) -> ("Numeric"=w397:dbl)  [unwired: 9 in, 1 out]
                n239 = local write "Test Slider"(w397) -> ()
                n240 = property on="Test Slider" class="Slide (strict)"("Visible"=TRUE, "Scale.Maximum"=100.0 ("Scale.Range:Maximum")) -> ()  [unwired: 2 in, 2 out]
                n241 = property on="Test Ring" class="Ring (strict)"("Visible"=FALSE) -> ()  [unwired: 2 in, 2 out]
              }
            }
          }
        }
        n242 = property on="Progress" class="Clust (strict)"("Visible"=FALSE) -> ()  [unwired: 2 in, 2 out]
      }
      event "Test Name": Mouse Enter {
        # "Populate the ring with the list of tests"
        n243 = event-data() -> ()  [unwired: 1 in, 1 out]
        n244 = call <vilib>:"NT Read String Array.vi"("Name"="/TestMode/TestList") -> ("String Array"=w406:string[])  [unwired: 9 in, 1 out]
        n245 = Build Array (concatenate)("Select the test to run...", w406) -> (w405:string[])
        n246 = property on="Test Name" class="Ring (strict)"("Strings []"=w405) -> ()  [unwired: 2 in, 2 out]
      }
      event "Test Name": Value Change {
        w408 = FALSE ("Visible")
        # "Tell the robot the test name to run"
        n247 = event-data() -> ("NewVal"=w412:u16)  [unwired: 1 in]
        n248 = property on="Test Name" class="Ring (strict)"() -> ("Strings []"=w413:string[])  [unwired: 2 in, 2 out]
        n249 = local write "Progress"(T6 {"Test Progress"=0, "Test Progress Text"=""} ("Progress")) -> ()
        n250 = Index Array(array=w413, index=w412) -> (element=w411:string)
        n251 = call <vilib>:"NT Write String.vi"("String"=w411, "Name"="/TestMode/TestName") -> ()  [unwired: 9 in, 1 out]
        n252 = property on="Progress" class="Clust (strict)"("Visible"=TRUE) -> ()  [unwired: 2 in, 2 out]
        n253 = property on="Motor" class="Clust (strict)"("Visible"=w408) -> ()  [unwired: 2 in, 2 out]
        n254 = property on="Test Slider" class="Slide (strict)"("Visible"=w408) -> ()  [unwired: 2 in, 2 out]
        n255 = property on="On/Off" class="Bool (strict)"("Visible"=w408) -> ()  [unwired: 2 in, 2 out]
        n256 = property on="Rev/Fwd" class="Clust (strict)"("Visible"=w408) -> ()  [unwired: 2 in, 2 out]
        n257 = property on="Test Ring" class="Ring (strict)"("Visible"=w408) -> ()  [unwired: 2 in, 2 out]
      }
      event "Select Auto": Mouse Enter {
        # "Populate the combo box with the list of autonomous options"
        n258 = event-data() -> ()  [unwired: 1 in, 1 out]
        n259 = call <vilib>:"NT Read String Array.vi"("Name"="Auto List") -> ("String Array"=w415:string[])  [unwired: 9 in, 1 out]
        n260 = property on="Select Auto" class="CmbBox"("Strings[]"=w415) -> ()  [unwired: 2 in, 2 out]
      }
      event "Select Auto": Value Change {
        # "User modified the Auto Selection. Write to NT variable so robot knows."
        n261 = event-data() -> ("NewVal"=w418:string)  [unwired: 1 in]
        n262 = call <vilib>:"NT Write String.vi"("String"=w418, "Name"="Auto Selector") -> ()  [unwired: 9 in, 1 out]
      }
      event "Command Selection": Value Change {
        # "Get the params and show in table"
        n263 = event-data() -> ("NewVal"=w424:i32)  [unwired: 1 in]
        n264 = property on="Command Selection" class="MCListbox (strict)"() -> ("ItemNames"=w422:string[][])  [unwired: 2 in, 2 out]
        n265 = call <vilib>:"WPI_DashboardUpdate Command Params.vi"("NewVal"=w424, "Commands"=w422, "Param Tbl"=w423) -> ()  [unwired: 8 in, 1 out]
      }
      event "Execute Command": Value Change {
        # "Started one, Unique ID holds\nresponse"
        n266 = event-data() -> ()  [unwired: 1 in, 1 out]
        n267 = property on="Command Selection" class="MCListbox (strict)"() -> ("ItemNames"=w435:string[][])  [unwired: 2 in, 2 out]
        n268 = Index Array(array=w435, index (row)="Command Selection", index (col)=0) -> (element=w433:string)
        n269 = call <vilib>:"Invoke Commands.vi"("Command Params"="Command Params", "Function Name"=w433) -> ("Params"=w429:u8, "Started"=w428:bool)  [unwired: 7 in, 1 out]
        n270 = Array Subset(array="Command Params", length (row)=w429) -> (w430:string[][])  [unwired: 3 in]
        n271 = Select(t="Executing" ("Cmd Status"), s=w428, f="" ("Cmd Status")) -> (s? t:f=→"Cmd Status":string)
      }
      event "Command Selection": Double Click {
        n272 = event-data() -> ("Row"=w443:i32)  [unwired: 1 in]
        n273 = property on="Command Selection" class="MCListbox (strict)"() -> ("ItemNames"=w446:string[][])  [unwired: 2 in, 2 out]
        n274 = local read "Command Params"() -> (w442:string[][])
        n275 = Index Array(array=w446, index (row)=w443, index (col)=0) -> (element=w444:string)
        n276 = call <vilib>:"Invoke Commands.vi"("Command Params"=w442, "Function Name"=w444) -> ("Params"=w441:u8, "Started"=w436:bool)  [unwired: 7 in, 1 out]
        n277 = Array Subset(array=w442, length (row)=w441) -> (w440:string[][])  [unwired: 3 in]
        n278 = Select(t="Executing" ("Cmd Status"), s=w436, f="" ("Cmd Status")) -> (s? t:f=w437:string)
        n279 = local write "Cmd Status"(w437) -> ()
      }
      event "CheckList": Double Click {
        # "Shift clears all"
        # "Update symbols on the listbox"
        n280 = event-data() -> ("PlatMods.Shift"=w448:bool, "Row"=w450:i32)  [unwired: 1 in]
        n281 = case shown="True" w448 {
          tunnel: w450 -> [w454 _]
          tunnel: 1 -> [w453 _]
          frame False {
            n282 = property on="CheckList" class="LstBox (strict)"() -> ("Item Symbols"=w452:i32[])  [unwired: 2 in, 2 out]
            n283 = Replace Array Subset(array=w452, new element=w453, index=w454) -> (w451:i32[])
            n284 = property on="CheckList" class="LstBox (strict)"("Item Symbols"=w451) -> ()  [unwired: 2 in, 2 out]
          }
          frame True {
            w455 = 0 ("Top Row")
            n285 = property on="CheckList" class="LstBox (strict)"() -> ("Number of Rows"=w457:u32)  [unwired: 2 in, 2 out]
            n286 = Initialize Array(0, w457) -> (w456:i32[])
            n287 = property on="CheckList" class="LstBox (strict)"("Top Row"=w455, "Value"=w455, "Item Symbols"=w456) -> ()  [unwired: 2 in, 2 out]
          }
        }
      }
      event "CheckList": Key Down {
        # "Update symbols on the listbox\nLeft and right keys check and uncheck"
        n288 = event-data() -> ("VKey"=w461:T20)  [unwired: 1 in]
        n289 = case shown="\"Left\", \"Right\"" w461 {
          selector: w461 -> [w466 _]
          tunnel: eventvkey."Left" ("VKey") -> [w464 _]
          frame "Left", "Right" {
            n290 = Equal?(x=w464, y=w466) -> (x = y?=w465:bool)
            n291 = Select(t=0, s=w465, f=1) -> (s? t:f=w467:i32)
            n292 = property on="CheckList" class="LstBox (strict)"() -> ("Item Symbols"=w470:i32[])  [unwired: 2 in, 2 out]
            n293 = Replace Array Subset(array=w470, new element=w467, index="CheckList") -> (w469:i32[])
            n294 = property on="CheckList" class="LstBox (strict)"("Item Symbols"=w469) -> ()  [unwired: 2 in, 2 out]
          }
          frame Default {
          }
        }
      }
      event "Motor.Enable": Value Change {
        # "When the test mode otor enable helper is set, update that\ntree row item's value"
        n295 = event-data() -> ("NewVal"=w476:bool)  [unwired: 1 in]
        n296 = Unbundle("Motor") -> ("Value"=w475:dbl)  [unwired: 1 out]
        n297 = Select(t=w475, s=w476, f=0.0) -> (s? t:f=w473:dbl)
        n298 = call <vilib>:"NT Write Number.vi"("Numeric"=w473, "Name"=w472) -> ()  [unwired: 9 in, 1 out]
      }
      event "Test Slider": Value Change {
        # "When the test mode slider helper is set, update that\ntree row item's value"
        n299 = event-data() -> ("NewVal"=w479:dbl)  [unwired: 1 in]
        n300 = call <vilib>:"NT Write Number.vi"("Numeric"=w479, "Name"=w480) -> ()  [unwired: 9 in, 1 out]
      }
      event "On/Off": Value Change {
        # "When the test mode on/off helper value is set, update that\ntree row item's value"
        n301 = event-data() -> ("NewVal"=w484:bool)  [unwired: 1 in]
        n302 = Boolean To (0,1)(Boolean=w484) -> (0, 1=w483:i16)
        n303 = call <vilib>:"NT Write Number.vi"("Numeric"=w483, "Name"=w482) -> ()  [unwired: 9 in, 1 out]
      }
      event "Rev/Fwd": Value Change {
        # "When the test mode helper value for relays is set, update that\ntree row item's value"
        n304 = event-data() -> ("NewVal.Forward"=w492:bool, "NewVal.Reverse"=w491:bool)  [unwired: 1 in]
        n305 = Boolean To (0,1)(Boolean=w492) -> (0, 1=w488:i16)
        n306 = Boolean To (0,1)(Boolean=w491) -> (0, 1=w490:i16)
        n307 = Negate(x=w490) -> (-x=w489:i16)
        n308 = Add(x=w488, y=w489) -> (x+y=w487:i16)
        n309 = call <vilib>:"NT Write Number.vi"("Numeric"=w487, "Name"=w486) -> ()  [unwired: 9 in, 1 out]
      }
      event "Test Ring": Value Change {
        # "When a test mode helper value is selected from the ring,\nset the tree item's variable to the string value"
        n310 = event-data() -> ("NewVal"=w496:u16)  [unwired: 1 in]
        n311 = property on="Test Ring" class="Ring (strict)"() -> ("Strings []"=w497:string[])  [unwired: 2 in, 2 out]
        n312 = Index Array(array=w497, index=w496) -> (element=w495:string)
        n313 = call <vilib>:"NT Write String.vi"("String"=w495, "Name"=w494) -> ()  [unwired: 9 in, 1 out]
      }
      event "Rec Mode": Value Change {
        # "Update globals for recording mode and path to read log from.\nClear when logging and let NetworkTables set path for vision to\nuse."
        n314 = event-data() -> ("NewVal"=w508:enum32{"Stop", "Record", "Playback"})  [unwired: 1 in]
        n315 = global write "WPI_DashboardLogging Global.vi" "Logging Filename"(path "") -> ()
        n316 = global write "WPI_DashboardLogging Global.vi" "Recording"(w508) -> ()
        n317 = case shown="\"Playback\"" w508 {
          tunnel: w507 -> [_ w510 w519]
          tunnel: [_ _ w518] -> w505
          tunnel: [_ _ w517] -> _
          tunnel: w503 -> [_ _ w515]
          tunnel: cluster{i32, i32} {-250, 170} -> [_ _ w514]
          tunnel: [_ _ T21 {"Image Size"=TRUE, "Image Type"=TRUE, "Pixel Value"=TRUE, "ROI Information"=TRUE, "Zoom Factor"=FALSE} ("Image Information Shown:All Elements")] -> w501
          tunnel: [_ _ TRUE ("Zoom Factor")] -> w500
          tunnel: w499 -> [_ _ w511]
          frame Default {
          }
          frame "Stop", "Record" {
            # "Place Window too"
            n318 = invoke class="VI" method="FP.Close"(reference=w510) -> (reference out=w509:refnum<vi>)  [unwired: 2 in, 2 out]
            n319 = invoke class="VI" method="Abort VI"(reference=w509) -> ()  [unwired: 2 in, 3 out]
          }
          frame "Playback" {
            n320 = call "Open Playback Panel.vi"("Offset"=w514, "DB VI Ref"=w515, "Playback in"=w519) -> ("Playback out"=w516:refnum<vi>)  [unwired: 8 in]
            n321 = register-events(w516, w511) -> (reference out=w518:refnum<event-registration>, error out=w517:errorcluster)  [unwired: 2 in]
          }
        }
        n322 = property on="Camera Image" class="ImageControl"("Image Information Shown"=w501, "Image Information Visible"=w500) -> ()  [unwired: 2 in, 2 out]
        n323 = call <vilib>:"WPI_DashboardNT Log FieldName Cache.vi"("Operation"=enum16{"Lookup/Add", "Index", "Clear"}."Clear") -> ()  [unwired: 8 in, 3 out]
      }
      event Panel Close {
        w521 = enum32{"Stop", "Record", "Playback"}."Stop" ("Rec Mode")
        # "Playback window has been closed, abort"
        n324 = event-data() -> ()  [unwired: 1 in, 4 out]
        n325 = local write "Rec Mode"(w521) -> ()
        n326 = global write "WPI_DashboardLogging Global.vi" "Recording"(w521) -> ()
      }
      event Panel Close {
        # "Abort playback window and ourself"
        n327 = event-data() -> ()  [unwired: 1 in, 4 out]
        n328 = invoke class="VI" method="FP.Close"(reference=w525) -> (reference out=w524:refnum<vi>)  [unwired: 2 in, 2 out]
        n329 = invoke class="VI" method="Abort VI"(reference=w524) -> (error out=w523:errorcluster)  [unwired: 2 in, 2 out]
        n330 = invoke class="VI" method="Abort VI"(error in=w523) -> ()  [unwired: 2 in, 3 out]
      }
      event User Event {
        n331 = event-data() -> ("IDs"=w532:cluster{"RPC field ID":u16, "Unique ID":u16}, "String"=w531:string)  [unwired: 1 in]
        n332 = Bundle("IDs"=w532, "String"=w531) -> (w530:T8)  [unwired: 1 in]
        n333 = call <vilib>:"Retrieve RPC Response.vi"("RPC Response"=w530) -> ("Output"=w528:string[][])  [unwired: 10 in]
        n334 = Build Array (concatenate)(w526, w528) -> (w527:string[][])
        n335 = local write "Command Params"(w527) -> ()
        n336 = local write "Cmd Status"("" ("Cmd Status")) -> ()
      }
      event "Tree": Double Click {
        n337 = event-data() -> ("PlatMods"=w536:T24, "Tag"=w535:string)  [unwired: 1 in]
        n338 = Unbundle(w536) -> ("Shift"=w534:bool)  [unwired: 4 out]
        n339 = Not(x=w534) -> (.not. x?=w533:bool)
        n340 = call <vilib>:"NT Update Persistence.vi"("Persistence"=w533, "Name"=w535) -> ()  [unwired: 9 in, 1 out]
      }
    }
  }
  n341 = while {
    tunnel: w64 -> [w539]
    i -> [w542]
    stop <- FALSE stop-if-true
    n342 = Wait (ms)(milliseconds to wait=u32 100) -> ()  [unwired: 1 out]
    n343 = case shown="\"Playback\"" "Rec Mode" {
      tunnel: w542 -> [_ _ w557]
      tunnel: [u32 2829099 ("Base Color") u32 11141120 ("Target Color") w546] -> w538
      frame "Stop", Default {
        # "Reset the color, extra updates don't cost much"
      }
      frame "Record" {
      }
      frame "Playback" {
        # "Playback"
        n344 = Quotient & Remainder(x=w557, y=u32 50 ("milliseconds to wait")) -> (x-y*floor(x/y)=w553:u32)  [unwired: 1 out]
        n345 = Divide(x=w553, y=u32 50 ("milliseconds to wait")) -> (x/y=w550:dbl)
        n346 = Multiply(x=6.283185307179586, y=w550) -> (x*y=w555:dbl)
        n347 = Sine(x=w555) -> (sin(x)=w554:dbl)
        n348 = Absolute Value(x=w554) -> (abs(x)=w547:dbl)
        n349 = call "Interpolate RGB Color.vi"("Proportion"=w547, "Target Color"=u32 30976, "Base Color"=u32 2829099) -> ("Result Color"=w546:u32)  [unwired: 8 in]
      }
    }
    n350 = property class="Pane"(reference=w539, "PaneColor"=w538) -> ()  [unwired: 1 in, 2 out]
  }
  n351 = local write "Dashboard Tab"(T2."Drive" ("Dashboard Tab")) -> ()
  n352 = property on="On/Off" class="Bool (strict)"("Visible"=w33) -> ()  [unwired: 2 in, 2 out]
  n353 = property on="Motor" class="Clust (strict)"("Visible"=w33) -> ()  [unwired: 2 in, 2 out]
  n354 = property on="Progress" class="Clust (strict)"("Visible"=w33) -> ()  [unwired: 2 in, 2 out]
  n355 = property on="Test Ring" class="Ring (strict)"("Visible"=w33) -> ()  [unwired: 2 in, 2 out]
  n356 = property on="Rev/Fwd" class="Clust (strict)"("Visible"=w33) -> ()  [unwired: 2 in, 2 out]
  n357 = local write "Command Selection"(u16 0 ("milliseconds to wait")) -> ()
  n358 = while {
    tunnel: u16 1741 ("timeout ms (25000)") -> [w559]
    stop <- FALSE stop-if-true
    n359 = TCP Create Listener(10:w559) -> (0:w558:errorcluster, 3:w560:refnum<k5>)  [unwired: 4 in, 1 out]
    n360 = case shown="No Error" w558 {
      selector: w558 -> [w562 _]
      tunnel: w560 -> [w563 _]
      frame No Error {
        n361 = while {
          tunnel: w563 -> [w566]
          tunnel: w562 -> [w565]
          stop <- FALSE stop-if-true
          n362 = TCP Wait On Listener(8:w565, 11:w566) -> (0:w567:errorcluster, 4:w568:refnum<k5>)  [unwired: 2 in, 3 out]
          n363 = local write "TCP"(w568) -> ()
          n364 = case shown="No Error" w567 {
            frame No Error {
            }
            frame Error {
              n365 = Wait (ms)(milliseconds to wait=u32 1000) -> ()  [unwired: 1 out]
            }
          }
        }
      }
      frame Error {
        n366 = Wait (ms)(milliseconds to wait=u32 1000) -> ()  [unwired: 1 out]
      }
    }
  }
  n367 = local write "Command Params"(string[][] [] ("Command Params")) -> ()
  n368 = global write "WPI_DashboardLogging Global.vi" "Recording"(w58) -> ()
  n369 = local write "Rec Mode"(w58) -> ()
  n370 = call <vilib>:"NT Write String.vi"("String"="Select Auto", "Name"="Auto Selector") -> ()  [unwired: 9 in, 1 out]
